vi "CLD 2 Elapsed Time Express FGV Exercise.vi"(7 "Express Timer FGV Enum":enum16{"Reset", "Read Status", "Set Auto Reset"}(ring), 8 "error in (no error)":errorcluster, 9 "Auto Reset (F)":bool, 10 "Time Target (s)":dbl=7.0) -> (0 "error out":errorcluster, 2 "Elapsed Time (s)":dbl, 3 "Time Has Elapsed":bool)   [LabVIEW 2019]
doc: "CLD 2 Exercise"
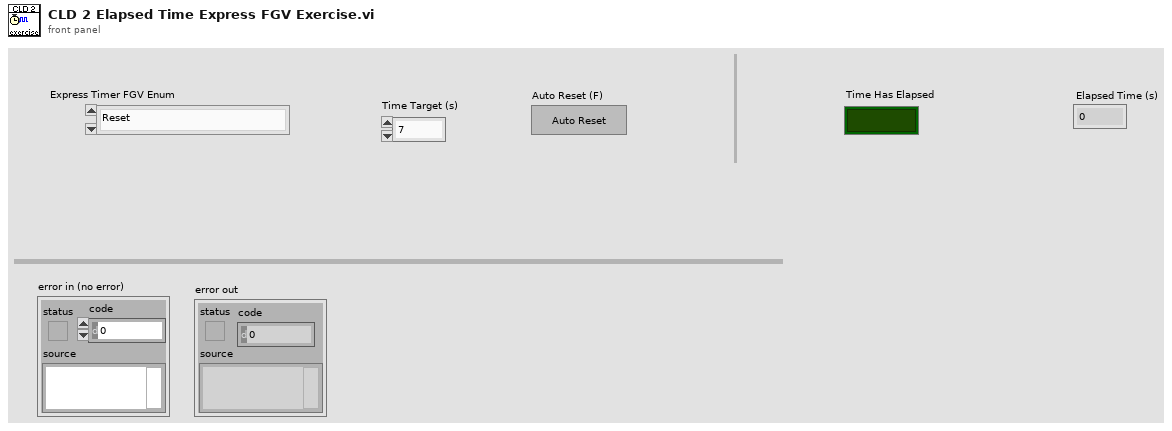
[diagram p1: front panel]
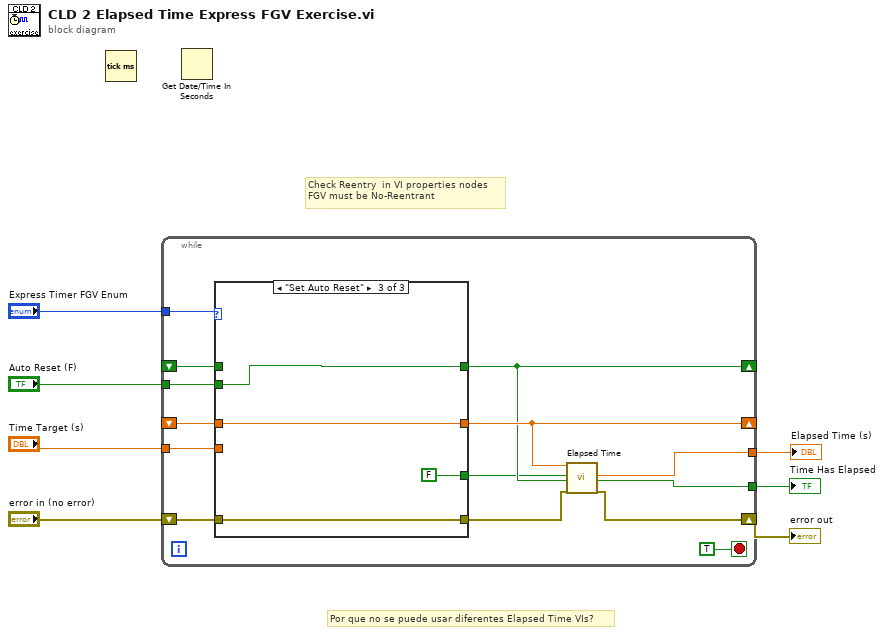
[diagram p0: block diagram]
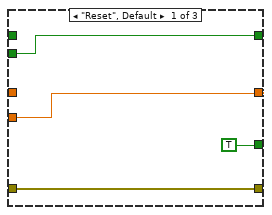
[diagram p2: hidden frame]
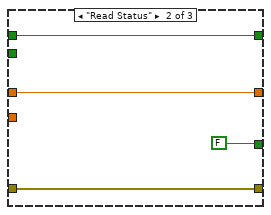
[diagram p3: hidden frame]
diagram:
  # "Check Reentry  in VI properties nodes\nFGV must be No-Reentrant"
  # "Por que no se puede usar diferentes Elapsed Time VIs?"
  n1 = Tick Count (ms)() -> ()  [unwired: 1 out]
  n2 = while {
    tunnel: "Express Timer FGV Enum" -> [w21]
    tunnel: "Time Target (s)" -> [w16]
    shift-right: [w13] -> w5
    shift-left: "error in (no error)" -> [w20]
    shift-right: [w10] -> _
    shift-left: _ -> [w18]
    tunnel: "Auto Reset (F)" -> [w17]
    shift-right: [w12] -> _
    shift-left: _ -> [w15]
    tunnel: [w11] -> w2
    tunnel: [w8] -> w1
    stop <- TRUE stop-if-true
    n3 = case shown="\"Set Auto Reset\"" w21 {
      tunnel: [w23 w27 w31] -> w14
      tunnel: w20 -> [w23 w27 w31]
      tunnel: w18 -> [_ w29 _]
      tunnel: [w24 w29 w33] -> w10
      tunnel: w17 -> [w24 _ w33]
      tunnel: w16 -> [w25 _ _]
      tunnel: [w25 w28 w32] -> w12
      tunnel: w15 -> [_ w28 w32]
      tunnel: [TRUE ("Auto Reset (F)") FALSE ("Auto Reset (F)") FALSE ("Auto Reset (F)")] -> w9
      frame "Reset", Default {
      }
      frame "Read Status" {
      }
      frame "Set Auto Reset" {
      }
    }
    n4 = call "Elapsed Time"("Time Target (s)"=w12, "Reset"=w9, "Auto Reset"=w10, "error in (no error)"=w14) -> ("Elapsed Time (s)"=w11:dbl, "Time has Elapsed"=w8:bool, "error out"=w13:errorcluster)  [unwired: 8 in, 5 out]
  }
  "error out" <- w5
  "Elapsed Time (s)" <- w2
  "Time Has Elapsed" <- w1
  n5 = Get Date/Time In Seconds() -> ()  [unwired: 1 out]
